vi "UHR-Fleezers Control (host) -Mau_stepping_gamma.vi"(0 "Tab Control":T5(tab)) -> ()   [LabVIEW 2013] (continued)
          frame #3 {
            # "Go to Bottom Dispensor"
            n244 = local read "Location Matrix"() -> (w465:string[][])
            n245 = Index Array(array=w465, index (row)=1) -> (element=w461:string[])  [unwired: 1 in]
            n246 = Decimate 1D Array(w461) -> (w459:string[], w457:string[], w455:string[])
            n247 = Concatenate Strings("1PA" ("Substring"), w459, "2PA" ("Substring"), w457, "3PA" ("Substring"), w455, "\r") -> (w463:string)
            n248 = local read "ESP Port"() -> (w462:refnum<visa-resource-name>)
            n249 = VISA Write(VISA resource name=w462, write buffer=w463) -> ()  [unwired: 1 in, 3 out]
          }
          frame #4 {
            n250 = Wait (ms)(milliseconds to wait=u32 200) -> ()  [unwired: 1 out]
          }
          frame #5 {
            # "Change the trajectory mode to Jog"
            n251 = local read "ESP Port"() -> (w467:refnum<visa-resource-name>)
            n252 = Concatenate Strings("1TJ3;\n2TJ3;\n3TJ3" ("Substring"), "\r") -> (w470:string)
            n253 = VISA Write(VISA resource name=w467, write buffer=w470) -> ()  [unwired: 1 in, 3 out]
          }
        }
      }
      event "Capture": Value Change {
        n254 = event-data() -> ()  [unwired: 1 in, 5 out]
        n255 = local read "Capture Locations"() -> (w471:i32)
        n256 = local read "Z Pos Pos"() -> (w472:string)
        n257 = local read "X Pos"() -> (w474:string)
        n258 = local read "Y Pos"() -> (w473:string)
        n259 = case shown="1" w471 {
          selector: w471 -> [w478 w485 w492 w499]
          tunnel: w474 -> [w481 w488 w495 w502]
          tunnel: w473 -> [w480 w487 w494 w501]
          tunnel: w472 -> [w479 w486 w493 w500]
          frame 0, Default {
            # "Capture Top Dispensor Location"
            n260 = local read "Location Matrix"() -> (w477:string[][])
            n261 = Build Array(w481, w480, w479) -> (w476:string[])
            n262 = Replace Array Subset(array=w477, new element=w476, index (row)=w478) -> (w475:string[][])  [unwired: 1 in]
            n263 = local write "Location Matrix"(w475) -> ()
          }
          frame 1 {
            # "Capture Bottom Dispensor Location"
            n264 = local read "Location Matrix"() -> (w484:string[][])
            n265 = Build Array(w488, w487, w486) -> (w483:string[])
            n266 = Replace Array Subset(array=w484, new element=w483, index (row)=w485) -> (w482:string[][])  [unwired: 1 in]
            n267 = local write "Location Matrix"(w482) -> ()
          }
          frame 2 {
            # "Capture Experimental Region Location"
            n268 = local read "Location Matrix"() -> (w491:string[][])
            n269 = Build Array(w495, w494, w493) -> (w490:string[])
            n270 = Replace Array Subset(array=w491, new element=w490, index (row)=w492) -> (w489:string[][])  [unwired: 1 in]
            n271 = local write "Location Matrix"(w489) -> ()
          }
          frame 3 {
            # "Capture Other Location"
            n272 = local read "Location Matrix"() -> (w498:string[][])
            n273 = Build Array(w502, w501, w500) -> (w497:string[])
            n274 = Replace Array Subset(array=w498, new element=w497, index (row)=w499) -> (w496:string[][])  [unwired: 1 in]
            n275 = local write "Location Matrix"(w496) -> ()
          }
        }
      }
      event "Save": Value Change {
        # "reshape Location Matrix to 1-D array to write"
        n276 = event-data() -> ()  [unwired: 1 in, 5 out]
        n277 = local read "Location Matrix"() -> (w506:string[][])
        n278 = local read "Location path"() -> (w503:path)
        n279 = Reshape Array(w506, 12) -> (w504:string[])
        n280 = Write to Text File(file (use dialog)=w503, text=w504) -> ()  [unwired: 2 in, 3 out]
      }
      event "Activate Joystick": Value Change {
        # "Change the trajectory mode to Jog"
        n281 = event-data() -> ()  [unwired: 1 in, 5 out]
        n282 = disable-structure shown="Disabled" {
          frame Disabled {
            n283 = case shown="True" "Activate Joystick" {
              frame False {
              }
              frame True {
                # "Change the trajectory mode to Jog"
                n284 = local read "ESP Port"() -> (w515:refnum<visa-resource-name>)
                n285 = Concatenate Strings("1TJ3;\n2TJ3;\n3TJ3" ("Substring"), "\r") -> (w512:string)
                n286 = VISA Write(VISA resource name=w515, write buffer=w512) -> ()  [unwired: 1 in, 3 out]
              }
            }
          }
          frame Enabled {
          }
        }
        n287 = local read "ESP Port"() -> (w507:refnum<visa-resource-name>)
        n288 = Concatenate Strings("1TJ3;\n2TJ3;\n3TJ3" ("Substring"), "\r") -> (w510:string)
        n289 = VISA Write(VISA resource name=w507, write buffer=w510) -> ()  [unwired: 1 in, 3 out]
      }
    }
  }
  n290 = disable-structure shown="Disabled" {
    disable-tunnel: w24 -> [w544 _]
    frame Disabled {
      w539 = T17 0 items=["Grayscale (U8)", "Grayscale (I16)", "Grayscale (SGL)", "Complex (CSG)", "RGB (U32)", "HSL (U32)", "RGB (U64)", "Grayscale (U16)"] ("Image Type")
      n291 = call <vilib>:"IMAQ Init.vi"("Interface Name"="img0") -> ("error out"=w541:errorcluster, "IMAQ Session Out"=w543:refnum<k11>)  [unwired: 9 in]
      n292 = call <vilib>:"IMAQ Grab Setup.vi"("error in (no error)"=w541, "IMAQ Session In"=w543) -> ("error out"=w537:errorcluster, "IMAQ Session Out"=w538:refnum<k11>)  [unwired: 8 in]
      n293 = call "IMAQ Create"("Image Name"="untitled", "Image Type"=w539) -> ("New Image"=w536:T3)  [unwired: 3 in, 1 out]
      n294 = call <vilib>:"Application Directory.vi"() -> ("Application Directory"=w523:path)
      n295 = Build Path(base path=w523, name or relative path="_trap_screen_positions") -> (appended path=w531:path)
      n296 = Open/Create/Replace File(file path (use dialog)=w531, operation (0:open)=T23."open or create", access (0:read/write)=enum16{"read/write", "read-only", "write-only"}."read/write") -> (refnum out=w533:refnum<file>)  [unwired: 3 in, 2 out]
      n297 = local read "Trap Sets"() -> (w525:u32)
      n298 = for "Load trap positions on video screen from file." {
        N: w525 -> [_]
        tunnel: [w551] -> w526
        tunnel: w533 -> [w550]
        tunnel: [w547] -> w522 mode=indexing
        w549 = 4
        n299 = for {
          N: w549 -> [_]
          tunnel: [w555] -> w551
          tunnel: w550 -> [w554]
          tunnel: w549 -> [w553]
          tunnel: [w552] -> w548 mode=indexing
          n300 = Read from Binary File(5:w553, 11:w554) -> (2:w552:i32, 3:w555:refnum<file>)  [unwired: 4 in, 2 out]
        }
        n301 = Array To Cluster(array=w548) -> (cluster=w547:T27)
      }
      n302 = node-c288() -> (w546:T24)  [unwired: 4 in]
      n303 = timed-loop "acquire video and stage position" {
        timing: w546 -> [_]
        timing-out: [_] -> w545
        tunnel: w538 -> [w574]
        tunnel: w537 -> [w573]
        tunnel: w536 -> [w572]
        tunnel: [w571] -> w518
        tunnel: [w568] -> w519
        tunnel: [w569] -> w517
        tunnel: w544 -> [_]
        shift-right: [w565] -> w535
        shift-left: w522 -> [w566]
        tunnel: w525 -> [w563]
        stop <- w570 stop-if-true
        n304 = node-c288() -> ()  [unwired: 1 in, 1 out]
        n305 = event shown="[0] Timeout" {
          selector: _ -> [_ _ _ _]
          dyn-events: _ -> [_ _ _ _]
          timeout: 10 -> [_ _ _ _]
          tunnel: w574 -> [w585 w600 w609 w628]
          tunnel: w573 -> [w584 w602 w607 w630]
          tunnel: w572 -> [w583 w601 w608 w629]
          tunnel: [w582 w600 w609 w628] -> w571
          tunnel: [w575 w604 FALSE FALSE] -> w570
          tunnel: [w579 w602 w607 w630] -> w569
          tunnel: [w578 w601 w608 w629] -> w568
          tunnel: "radius" -> [_ _ w614 _]
          tunnel: w566 -> [w576 w603 w612 _]
          tunnel: [w576 w603 w613 cluster{i32, i32, i32, i32}[] []] -> w565
          tunnel: w563 -> [_ _ w605 _]
          event Timeout {
            n306 = event-data() -> ()  [unwired: 1 in, 2 out]
            n307 = call <vilib>:"IMAQ Grab Acquire.vi"("error in (no error)"=w584, "Image In"=w583, "IMAQ Session In"=w585) -> ("error out"=w580:errorcluster, "Image Out"=w581:T3, "IMAQ Session Out"=w582:refnum<k11>)  [unwired: 5 in, 1 out]
            n308 = case shown="True" "trap\nmarkers?" {
              tunnel: w576 -> [_ w593]
              tunnel: w581 -> [w587 w592]
              tunnel: w580 -> [w586 w591]
              tunnel: [w586 w590] -> w579
              tunnel: [w587 w588] -> w578
              frame False {
              }
              frame True {
                n309 = for {
                  tunnel: w593 -> [w599] mode=indexing
                  shift-right: [w597] -> w588
                  shift-left: w592 -> [w598]
                  tunnel: w591 -> [w596]
                  tunnel: [w595] -> w590
                  tunnel: u32 16711680 ("Color") -> [w594]
                  n310 = call "IMAQ Overlay Oval"("Color"=w594, "error in (no error)"=w596, "Bounding Rectangle"=w599, "Image"=w598) -> ("error out"=w595:errorcluster, "Image Out"=w597:T3)  [unwired: 6 in]
                }
              }
            }
            "Primary Video Display" <- w578
            n311 = Unbundle By Name(w580) -> ("status"=w575:bool)
          }
          event "Stop All": Value Change {
            n312 = event-data() -> ()  [unwired: 1 in, 5 out]
            n313 = local read "Stop All"() -> (w604:bool)
          }
          event "Primary Video Display": Mouse Down {
            n314 = event-data() -> ()  [unwired: 1 in, 7 out]
            n315 = Array Size(array=w612) -> (size(s)=w611:i32)
            n316 = Less?(x=w611, y=w605) -> (x < y?=w610:bool)
            n317 = case shown="True" w610 {
              tunnel: w614 -> [_ w624]
              tunnel: w612 -> [w615 w618]
              tunnel: [w615 w617] -> w613
              frame False {
              }
              frame True {
                n318 = property on="Primary Video Display" class="ImageControl"() -> ("Last Mouse Position"=w616:cluster{"X":i32, "Y":i32})  [unwired: 2 in, 2 out]
                n319 = Unbundle By Name(w616) -> ("X"=w626:i32, "Y"=w625:i32)
                n320 = Add(x=w625, y=w624) -> (x+y=w622:i32)
                n321 = Subtract(x=w625, y=w624) -> (x-y=w620:i32)
                n322 = Add(x=w626, y=w624) -> (x+y=w621:i32)
                n323 = Subtract(x=w626, y=w624) -> (x-y=w623:i32)
                n324 = Bundle(w623, w622, w621, w620) -> (w619:cluster{i32, i32, i32, i32})  [unwired: 1 in]
                n325 = Build Array (concatenate)(w618, w619) -> (w617:T28)
              }
            }
          }
          event "clear markers": Value Change {
            n326 = event-data() -> ()  [unwired: 1 in, 5 out]
          }
        }
        n327 = node-c288() -> ()  [unwired: 1 in, 1 out]
      }
      n328 = node-c288(w545) -> ()  [unwired: 1 out]
      n329 = Set File Position(offset (in bytes) (0)=i64 0, refnum=w526, from (0:start)=enum16{"start", "end", "current"}."start") -> (refnum out=w527:refnum<file>)  [unwired: 1 in, 1 out]
      n330 = for "Write trap positions to file so they can be remembered\nwhen program is removed from memory" {
        tunnel: w535 -> [w559] mode=indexing
        tunnel: [w557] -> w534
        tunnel: w527 -> [w556]
        n331 = Cluster To Array(cluster=w559) -> (array=w558:i32[])
        n332 = for {
          tunnel: w558 -> [w562] mode=indexing
          tunnel: [w561] -> w557
          tunnel: w556 -> [w560]
          n333 = Write to Binary File(file (use dialog)=w560, data=w562) -> (refnum out=w561:refnum<file>)  [unwired: 4 in, 2 out]
        }
      }
      n334 = Close File(refnum=w534) -> ()  [unwired: 1 in, 2 out]
      n335 = call "IMAQ Dispose"("Image"=w519, "error in (no error)"=w517) -> ("error out"=w516:errorcluster)  [unwired: 4 in]
      n336 = call <vilib>:"IMAQ Stop.vi"("error in (no error)"=w516, "IMAQ Session In"=w518) -> ("error out"=w520:errorcluster, "IMAQ Session Out"=w521:refnum<k11>)  [unwired: 8 in]
      n337 = call <vilib>:"IMAQ Close.vi"("error in (no error)"=w520, "IMAQ Session In"=w521) -> ()  [unwired: 9 in, 1 out]
    }
    frame Enabled {
    }
  }
  n338 = disable-structure shown="Enabled" {
    disable-tunnel: [w637 _] -> w35
    disable-tunnel: w24 -> [w636 _]
    frame Enabled {
      n339 = node-c288() -> (w639:T24)  [unwired: 4 out]
      n340 = timed-loop "Rough control of MCL mirror stage (debugging)" {
        tunnel: w636 -> [w642]
        tunnel: [w641] -> w637
        timing: w639 -> [_]
        timing-out: [_] -> w638
        stop <- w641 stop-if-true
        n341 = node-c288() -> ()  [unwired: 2 out]
        n342 = case shown="1" "MCL Mode" {
          tunnel: w642 -> [_ w645 w692]
          frame 0, Default {
            # "manual positioning"
          }
          frame 1 {
            # "sinusoidal wave"
            n343 = node-c288() -> (w647:T24)  [unwired: 4 out]
            n344 = timed-loop "Oscillate MCL mirror" {
              timing: w647 -> [_]
              timing-out: [_] -> w646
              tunnel: w645 -> [w686]
              i -> [w685]
              stop <- w648 stop-if-true
              n345 = node-c288() -> (w684:i64)  [unwired: 1 out]
              n346 = Multiply(x="AO1", y=32767.0) -> (x*y=w680:dbl)
              n347 = Multiply(x="AO2", y=32767.0) -> (x*y=w675:dbl)
              n348 = Divide(x=w680, y=10.0) -> (x/y=w681:dbl)
              n349 = Divide(x=w675, y=10.0) -> (x/y=w676:dbl)
              n350 = To Word Integer(number=w681) -> (16bit integer=w673:i16)
              n351 = To Word Integer(number=w676) -> (16bit integer=w672:i16)
              n352 = Divide(x=w684, y=i64 1000) -> (x/y=w655:dbl)
              n353 = Multiply(x=w655, y=w685) -> (x*y=w666:dbl)
              n354 = Multiply(x="Osc. freq. (Hz) 2", y=6.283185307179586) -> (x*y=w667:dbl)
              n355 = Multiply(x=w667, y=w666) -> (x*y=w665:dbl)
              n356 = Sine(x=w665) -> (sin(x)=w664:dbl)
              n357 = Multiply(x=w664, y="Osc. amp. (V)") -> (x*y=w662:dbl)
              n358 = Add(x=w662, y="Osc. center (V)") -> (x+y=w660:dbl)
              n359 = Divide(x=w660, y=10.0) -> (x/y=w658:dbl)
              n360 = Multiply(x=w658, y=32767.0) -> (x*y=w653:dbl)
              n361 = Select(t=w653, s="Scan axis", f=w673) -> (s? t:f=w671:dbl)
              n362 = Select(t=w672, s="Scan axis", f=w653) -> (s? t:f=w670:dbl)
              n363 = local read "MCL Mode"() -> (w652:u16)
              n364 = Not Equal?(x=w652, y=u16 1) -> (x != y?=w649:bool)
              n365 = local read "Stop All"() -> (w650:bool)
              n366 = xnode "Read/Write Control"("FPGA VI Reference In"=w686, "AO1"=w671, "AO2"=w670) -> ()  [unwired: 1 in, 2 out]
              n367 = Compound Arithmetic op=OR(w650, w649) -> (w648:bool)
              n368 = node-c288() -> ()  [unwired: 2 out]
            }
            n369 = node-c288(w646) -> ()  [unwired: 1 out]
          }
          frame 2 {
            # "linear scan"
            n370 = case shown="True" "Start Scan" {
              tunnel: w692 -> [_ w704]
              frame False {
              }
              frame True {
                n371 = Subtract(x="End (V)", y="Begin (V)") -> (x-y=w700:dbl)
                n372 = Decrement(x="N Points") -> (x-1=w699:dbl)
                n373 = Divide(x=w700, y=w699) -> (x/y=w697:dbl)
                n374 = for {
                  N: "N Points" -> [_]
                  tunnel: "Begin (V)" -> [w717]
                  tunnel: w704 -> [w709]
                  tunnel: [w708] -> w703 mode=indexing
                  tunnel: w697 -> [w707]
                  tunnel: [w705] -> w696 mode=indexing
                  i -> [w716]
                  n375 = Multiply(x=w707, y=w716) -> (x*y=w715:dbl)
                  n376 = Add(x=w717, y=w715) -> (x+y=w712:dbl)
                  n377 = local read "Scan axis"() -> (w706:bool)
                  n378 = local read "AO1"() -> (w714:dbl)
                  n379 = local read "AO2"() -> (w713:dbl)
                  n380 = Select(t=w712, s=w706, f=w714) -> (s? t:f=w711:dbl)
                  n381 = Select(t=w713, s=w706, f=w712) -> (s? t:f=w710:dbl)
                  n382 = flat-sequence {
                    tunnel: w711 -> [w721]
                    tunnel: w710 -> [w720]
                    tunnel: w709 -> [w718]
                    tunnel: [w731] -> w708
                    tunnel: [w730] -> w705
                    frame #0 {
                      w724 = 10.0 ("y")
                      w719 = 32767.0 ("y")
                      n383 = Multiply(x=w721, y=w719) -> (x*y=w727:dbl)
                      n384 = Multiply(x=w720, y=w719) -> (x*y=w725:dbl)
                      n385 = Divide(x=w727, y=w724) -> (x/y=w728:dbl)
                      n386 = Divide(x=w725, y=w724) -> (x/y=w726:dbl)
                      n387 = To Word Integer(number=w728) -> (16bit integer=w722:i16)
                      n388 = To Word Integer(number=w726) -> (16bit integer=w723:i16)
                      n389 = xnode "Read/Write Control"("FPGA VI Reference In"=w718, "AO1"=w722, "AO2"=w723) -> ()  [unwired: 1 in, 2 out]
                    }
                    frame #1 {
                      n390 = Wait (ms)(milliseconds to wait="DAQ Delay (ms)") -> ()  [unwired: 1 out]
                    }
                    frame #2 {
                      n391 = local read "Slow mean"() -> (w731:dbl)
                      n392 = local read "Sigma"() -> (w730:dbl)
                    }
                  }
                }
                n393 = Bundle("Begin (V)"="Begin (V)", w697, w703) -> (→"MCL Scan":cluster{"Begin (V)":dbl, dbl, dbl[]})  [unwired: 1 out]
                n394 = Bundle("Begin (V)"="Begin (V)", w697, w696) -> (→"MCL Scan 2":cluster{"Begin (V)":dbl, dbl, dbl[]})  [unwired: 1 out]
              }
            }
          }
        }
        n395 = local read "Stop All"() -> (w641:bool)
        n396 = node-c288() -> ()  [unwired: 2 out]
      }
      n397 = node-c288(w638) -> ()  [unwired: 1 out]
    }
    frame Disabled {
    }
  }
  n398 = node-c288(2 ("Processor")) -> (w15:T24)  [unwired: 3 in]
  n399 = node-c288() -> (w69:T24)  [unwired: 4 in]
  n400 = timed-loop "Control parameters (event loop)" {
    tunnel: w24 -> [w737]
    shift-right: [w736] -> _
    shift-left: errorcluster {"status"=FALSE, "code"=0, "source"=""} ("error out") -> [w735]
    tunnel: [w734] -> w37
    timing: w15 -> [_]
    timing-out: [_] -> w14
    stop <- w734 stop-if-true
    n401 = node-c288() -> ()  [unwired: 1 in, 1 out]
    n402 = event shown="[7] \"Simulate motor gamma distribution\": Value Change" {
      selector: _ -> [_ _ _ _ _ _ _ _ _ _ _ _ _ _ _ _ _ _ _ _ _ _ _ _ _ _ _ _ _ _ _ _ _ _ _ _ _ _ _ _ _ _ _ _ _ _ _ _ _ _ _ _ _ _ _ _ _]
      dyn-events: _ -> [_ _ _ _ _ _ _ _ _ _ _ _ _ _ _ _ _ _ _ _ _ _ _ _ _ _ _ _ _ _ _ _ _ _ _ _ _ _ _ _ _ _ _ _ _ _ _ _ _ _ _ _ _ _ _ _ _]
      timeout: _ -> [_ _ _ _ _ _ _ _ _ _ _ _ _ _ _ _ _ _ _ _ _ _ _ _ _ _ _ _ _ _ _ _ _ _ _ _ _ _ _ _ _ _ _ _ _ _ _ _ _ _ _ _ _ _ _ _ _]
      tunnel: w737 -> [w775 _ _ _ w812 _ w834 w864 _ w951 _ _ _ w994 _ _ w1037 w1043 w1048 w1054 w1090 w1108 w1115 w1133 w1144 w1155 w1166 w1177 w1188 w1206 w1212 w1306 _ w1315 w1353 _ w1388 w1392 w1403 w1407 w1411 _ w1419 _ _ _ _ _ w1555 _ w1572 w1575 w1584 w1587 w1591 _ w1608]
      tunnel: [w774 _ _ _ w802 _ w833 w863 _ w914 _ w959 _ w973 _ _ w1036 w1039 w1045 w1051 w1089 w1106 w1114 w1127 w1138 w1149 w1160 w1171 w1182 w1204 w1211 w1304 _ w1313 w1351 _ w1386 w1390 w1393 w1405 w1409 _ w1417 _ _ _ _ _ w1553 _ _ _ _ _ _ _ _] -> w736
      tunnel: w735 -> [w773 _ _ _ w811 _ w832 w862 _ w946 _ w959 _ w993 _ _ w1035 w1038 w1044 w1050 w1088 w1107 w1113 w1132 w1143 w1154 w1165 w1176 w1187 w1205 w1210 w1305 _ w1314 w1352 _ w1387 w1391 w1402 w1406 w1410 _ w1418 _ _ _ _ _ w1554 _ w1571 w1574 w1583 w1586 w1590 _ w1607]
      tunnel: [_ _ _ _ _ _ _ _ _ _ _ w958 _ _ _ _ _ _ _ _ _ _ _ _ _ _ _ _ _ _ _ _ _ _ _ _ _ _ _ _ _ _ _ _ _ _ _ _ _ _ _ _ _ _ _ _ _] -> w734
      tunnel: [_ _ _ _ _ _ _ _ "Round T1 X" _ _ _ _ _ _ _ _ _ _ _ _ _ _ _ _ _ _ _ _ _ _ _ _ _ _ _ _ _ _ _ _ _ _ _ _ _ _ _ _ _ _ _ _ _ _ _ _] -> _
      tunnel: [_ _ _ "Adjust Scale\nto Mean" _ _ _ _ _ _ _ _ _ _ _ _ _ _ _ _ _ _ _ _ _ _ _ _ _ _ _ _ _ _ _ _ _ _ _ _ _ _ _ _ _ _ _ _ _ _ _ _ _ _ "Set SP to Reading" _ _] -> _
      tunnel: [_ _ _ _ _ _ _ _ _ _ "Round T2 X" _ "Delayed Interlace Start" _ _ _ _ _ _ _ _ _ _ _ _ _ _ _ _ _ _ _ _ _ _ _ _ _ _ _ _ _ _ _ _ _ _ _ _ _ _ _ _ _ _ _ _] -> _
      event "AI Count (ticks)", "Sets to FIFO (Traps)", "Save ave N", "FPGA Ave.", "# Samples/channel", "N sets to save": Value Change {
        # "So that if 'Save ave N' is updated, the AOD scanning code updates too."
        n403 = event-data() -> ()  [unwired: 6 out]
        n404 = local read "AI Count (ticks)"() -> (w755:u32)
        n405 = Boolean To (0,1)(Boolean="Sets to FIFO (Traps)") -> (0, 1=w765:cluster{"Set 1":i16, "Set 2":i16, "Set 3":i16})
        n406 = xnode "Read/Write Control"("FPGA VI Reference In"=w775, "error in"=w773, "ai count"=w755, "AI1 Sets to FIFO"="Sets to FIFO (Traps)", "N of AI1 Int Acq Sets"="N Acq Sets (Traps + Fl.)") -> ("error out"=w774:errorcluster)  [unwired: 1 out]
        n407 = Cluster To Array(cluster=w765) -> (array=w764:i16[])
        n408 = To Unsigned Long Integer(number=w764) -> (unsigned 32bit integer=w744:u32[])
        n409 = local read "Scan steps (AOD)"() -> (w766:u64)
        n410 = Multiply(x=w755, y="N Acq Sets (Traps + Fl.)") -> (x*y=w753:u32)
        n411 = Divide(x=40000000.0, y=w755) -> (x/y=w747:dbl)
        "AI rate (Hz)" <- w747
        "Ave. Rate (Hz)" <- w747
        n412 = Add Array Elements(numeric array=w744) -> (sum=w756:u32)
        "Trap Sets" <- w756
        n413 = Reciprocal(x=w747) -> (1/x=→"Ave. Period (s)":dbl)
        n414 = property on="Scan steps (AOD)" class="DigNum (strict)"("Val(Sgnl)"=w766) -> ()  [unwired: 2 in, 2 out]
        n415 = Divide(x=w747, y="N Acq Sets (Traps + Fl.)") -> (x/y=w770:dbl)
        "Data Rate (Hz)" <- w770
        n416 = Reciprocal(x=w770) -> (1/x=→"Data Period (s)":dbl)
        n417 = local read "Save ave N"() -> (w769:dbl)
        n418 = Divide(x=w770, y=w769) -> (x/y=w768:dbl)
        "Save Data Rate (Hz)" <- w768
        n419 = Reciprocal(x=w768) -> (1/x=→"Save Data Period (s)":dbl)
        n420 = Multiply(x=w753, y="# Samples/trap") -> (x*y=w751:u32)
        "Counts/DMA" <- w751
        n421 = property on="Trap Disp. Downsample" class="DigNum (strict)"("Maximum"="# Samples/trap") -> ()  [unwired: 2 in, 2 out]
        n422 = Multiply(x=w756, y="# Samples/trap") -> (x*y=w745:u32)
        "# Samples/channel" <- w745
        n423 = Multiply(x=w745, y=u32 8) -> (x*y=→"Trap AI Elements/DMA read":u32)
        n424 = local read "APD Int. Count"() -> (w752:u32)
        n425 = Multiply(x=w745, y=u32 3) -> (x*y=→"Trap Pos Elements/DMA read":u32)
        n426 = Divide(x=w751, y=w752) -> (x/y=w742:dbl)
        "APD Samples/FIFO Acq." <- w742
        n427 = Divide(x=w751, y=40000000.0) -> (x/y=w749:dbl)
        "DMA Update Period (s)" <- w749
        n428 = Multiply(x=2.0, y=w742) -> (x*y=→"APD Elements/DMA read":dbl)
        n429 = property on="APD Disp. Downsample" class="DigNum (strict)"("Maximum"=w742) -> ()  [unwired: 2 in, 2 out]
        n430 = local read "N sets to save"() -> (w762:u32)
        n431 = Multiply(x=w749, y=w762) -> (x*y=→"Total Time (s)":dbl)
        "FPGA Averaging" <- FALSE ("FPGA Averaging")
      }
      event "Rescale on Mean": Value Change {
        n432 = event-data() -> ()  [unwired: 7 out]
        n433 = And(x=FALSE, y="Rescale on Mean") -> (x .and. y?=w777:bool)
        n434 = local write "Rescale on Mean"(w777) -> ()
        n435 = local read "Bead Mean (nm)"() -> (w782:dbl)
        n436 = Add(x="Amplitude (nm)", y=w782) -> (x+y=w780:dbl)
        n437 = Subtract(x=w782, y="Amplitude (nm)") -> (x-y=w779:dbl)
        n438 = property on="Bead Separation" class="WFChart (strict)"("YScale.Minimum"=w779) -> ()  [unwired: 2 in, 2 out]
        n439 = property on="Bead Separation" class="WFChart (strict)"("YScale.Maximum"=w780) -> ()  [unwired: 2 in, 2 out]
      }
      event "Detector Type": Value Change {
        n440 = event-data() -> ()  [unwired: 7 out]
        n441 = local read "AI labels"() -> (w783:string[])
        n442 = property on="High Res. Display" class="Ring (strict)"("Strings []"=w783) -> ()  [unwired: 2 in, 2 out]
        n443 = Build Array (concatenate)(w783, "none") -> (w784:string[])
        n444 = property on="FFT 1 Choice 1" class="Ring (strict)"("Strings []"=w784) -> ()  [unwired: 2 in, 2 out]
        n445 = property on="FFT 1 Choice 2" class="Ring (strict)"("Strings []"=w784) -> ()  [unwired: 2 in, 2 out]
        n446 = property on="FFT 2 Choice 1" class="Ring (strict)"("Strings []"=w784) -> ()  [unwired: 2 in, 2 out]
        n447 = property on="FFT 2 Choice 2" class="Ring (strict)"("Strings []"=w784) -> ()  [unwired: 2 in, 2 out]
        n448 = Bundle("APD 1", "APD 2") -> (w787:cluster{string, string})  [unwired: 1 out]
        n449 = Cluster To Array(cluster=w787) -> (array=w785:string[])
        n450 = Build Array (concatenate)(w785, w784) -> (w789:string[])
        n451 = Array Size(array=w789) -> (size(s)=w790:i32)
        n452 = property on="Signals to Plot" class="LstBox (strict)"("Item Names"=w789) -> ()  [unwired: 2 in, 2 out]
        n453 = property on="Signals to Plot" class="LstBox (strict)"("Number of Rows"=w790) -> ()  [unwired: 2 in, 2 out]
        n454 = property on="All Signals" class="WFChart (strict)"("LegNumRows"=w790) -> ()  [unwired: 2 in, 2 out]
      }
      event "Adjust Scale\nto Mean": Value Change {
        n455 = event-data() -> ()  [unwired: 7 out]
        n456 = local read "APD 1 Rate (Hz)"() -> (w799:dbl)
        n457 = Multiply(x=1000.0, y="Above (kHz)") -> (x*y=w797:dbl)
        n458 = Multiply(x=1000.0, y="Below (kHz)") -> (x*y=w795:dbl)
        n459 = Add(x=w797, y=w799) -> (x+y=w792:dbl)
        n460 = Subtract(x=w799, y=w795) -> (x-y=w793:dbl)
        n461 = property on="APD Chart" class="WFChart (strict)"("YScale.Minimum"=w793) -> ()  [unwired: 2 in, 2 out]
        n462 = property on="APD Chart" class="WFChart (strict)"("YScale.Maximum"=w792) -> ()  [unwired: 2 in, 2 out]
      }
      event "Phase adj. (AI1)", "+ phase (AI1)", "- phase (AI1)": Value Change {
        n463 = event-data() -> ()  [unwired: 7 out]
        n464 = Negate(x="Phase adj. (AI1)") -> (-x=w809:i16)
        n465 = Select(t=w809, s="- phase (AI1)", f="Phase adj. (AI1)") -> (s? t:f=w808:i16)
        n466 = xnode "Read/Write Control"("FPGA VI Reference In"=w812, "error in"=w811, "Phase count adjustment"=w808) -> ("FPGA VI Reference Out"=w807:T19, "error out"=w806:errorcluster)
        n467 = Or(x="- phase (AI1)", y="+ phase (AI1)") -> (x .or. y?=w803:bool)
        n468 = xnode "Read/Write Control"("FPGA VI Reference In"=w807, "error in"=w806, "+ phase"=w803) -> ("error out"=w802:errorcluster)  [unwired: 1 out]
      }
      event "Signals to Plot": Double Click {
        w815 = u32 9868950 ("Color Box")
        n469 = event-data() -> ("Row"=w817:i32)  [unwired: 9 out]
        n470 = property on="All Signals" class="WFChart (strict)"("Active Plot"=w817) -> (error out=w828:errorcluster)  [unwired: 2 in, 1 out]
        n471 = property on="All Signals" class="WFChart (strict)" props=["Plot", "Visible?", "Plot", "Plot Color"](error in=w828) -> (error out=w827:errorcluster, "Plot.Visible?"=w826:bool)  [unwired: 1 in, 2 out]
        n472 = Select(t=FALSE ("Plot.Visible"), s=w826, f=TRUE ("Plot.Visible")) -> (s? t:f=w821:bool)
        n473 = property on="All Signals" class="WFChart (strict)"(error in=w827, "Plot.Visible?"=w821) -> (error out=w823:errorcluster)  [unwired: 1 in, 1 out]
        n474 = property on="All Signals" class="WFChart (strict)"(error in=w823) -> (error out=w818:errorcluster, "Plot.Plot Color"=w822:u32)  [unwired: 1 in, 1 out]
        n475 = property on="Signals to Plot" class="LstBox (strict)"(error in=w818, "Active Row"=w817) -> (error out=w816:errorcluster)  [unwired: 1 in, 1 out]
        n476 = Select(t=w822, s=w821, f=u32 0) -> (s? t:f=w819:u32)
        n477 = property on="Signals to Plot" class="LstBox (strict)"(error in=w816, "CellFontColor"=w819, "SelColor"=w815, "CellBG"=w815, "CellFontSize"=u32 20 ("Active Row:Cell Font:Size"), "CellFontBold"=TRUE ("Active Row:Cell Font:Bold")) -> ()  [unwired: 1 in, 2 out]
      }
      event "BD 1 Frequency 1 (MHz)", "BD 1 Frequency 2 (MHz)", "BD 1 Frequency 3 (MHz)", "BD 2 Frequency 1 (MHz)", "BD 2 Frequency 2 (MHz)", "BD 2 Frequency 3 (MHz)", "Trap Delta (MHz)": Value Change {
        # "anytime one of the frequencies is changed, write it to the RF board UNLESS Set 2 is being oscillated. The oscillation\nscript writes the frequencies to the RF board."
        n478 = event-data() -> ("CtlRef"=w831:refnum<vi>)  [unwired: 6 out]
        n479 = control-ref of="Trap Delta (MHz)"() -> (w830:refnum<vi>)
        n480 = Equal?(x=w830, y=w831) -> (x = y?=w829:bool)
        n481 = case shown="False" "Oscillate Set 2" {
          tunnel: w834 -> [w857 _]
          tunnel: [w856 w860] -> w833
          tunnel: w832 -> [w855 w860]
          tunnel: w829 -> [w842 _]
          frame False {
            w836 = 80
            n482 = local read "BD 1 Frequency 2 (MHz)"() -> (w844:dbl)
            n483 = Divide(x="Trap Delta (MHz)", y=2) -> (x/y=w838:dbl)
            n484 = Subtract(x=w836, y=w838) -> (x-y=w837:dbl)
            n485 = local write "BD 1 Frequency 1 (MHz)"(w837) -> ()
            n486 = Add(x=w836, y=w838) -> (x+y=w843:dbl)
            n487 = Select(t=w843, s=w842, f=w844) -> (s? t:f=w841:dbl)
            n488 = local read "Y RF Frequency Limits (MHz)"() -> (w845:T16)
            n489 = local read "X RF Frequency Limits (MHz)"() -> (w846:T16)
            n490 = local read "BD 1 Frequency 3 (MHz)"() -> (w858:dbl)
            n491 = local write "BD 1 Frequency 2 (MHz)"(w841) -> ()
            n492 = local read "BD 2 Frequency 1 (MHz)"() -> (w849:dbl)
            n493 = local read "BD 2 Frequency 2 (MHz)"() -> (w848:dbl)
            n494 = local read "BD 2 Frequency 3 (MHz)"() -> (w859:dbl)
            n495 = call "set RF board frequency - interlace.vi"("Board 2 Frequency Limits"=w845, "Board 1 Frequency Limits"=w846, "error in"=w855, "FPGA VI Reference In"=w857, "Board 2 Frequency 3 (MHz)"=w859, "Board 1 Frequency 3 (MHz)"=w858, "Board 2 Frequency 2 (MHz)"=w848, "Board 2 Frequency 1 (MHz)"=w849, "Board 1 Frequency 2 (MHz)"=w841, "Board 1 Frequency 1  (MHz)"=w837) -> ("error out"=w856:errorcluster)  [unwired: 1 out]
            n496 = Subtract(x=w849, y=w848) -> (x-y=w853:dbl)
            n497 = Subtract(x=w841, y=w837) -> (x-y=w854:dbl)
            n498 = Square(x=w853) -> (x^2=w851:dbl)
            n499 = Square(x=w854) -> (x^2=w852:dbl)
            n500 = Add(x=w852, y=w851) -> (x+y=w850:dbl)
            n501 = Square Root(x=w850) -> (sqrt(x)=w847:dbl)
            n502 = local write "Trap Delta (MHz)"(w847) -> ()
            n503 = property on="Initial delta (MHz)" class="DigNum (strict)"("Val(Sgnl)"=w847) -> ()  [unwired: 2 in, 2 out]
          }
          frame True {
          }
        }
      }
      event "Simulate motor gamma distribution": Value Change {
        n504 = event-data() -> ()  [unwired: 7 out]
        n505 = flat-sequence {
          tunnel: w864 -> [w867]
          tunnel: w862 -> [w865]
          tunnel: [w866] -> w861
          tunnel: [w910] -> w863
          tunnel: w861 -> [w910]
          frame #0 {
            n506 = while {
              tunnel: w867 -> [w908]
              tunnel: [w907] -> w866
              tunnel: w865 -> [w906]
              i -> [w890]
              stop <- w892 stop-if-true
              n507 = Divide(x="Backtrack probability", y=100) -> (x/y=w883:dbl)
              n508 = Random Number (0-1)() -> (number: 0 to 1=w882:dbl)
              n509 = Greater?(x=w882, y=w883) -> (0:w881:bool)
              n510 = Select(t=1, s=w881, f=-1) -> (s? t:f=w878:i32)
              n511 = local read "BD 1 Frequency 2 (MHz)"() -> (w894:dbl)
              n512 = Multiply(x=w878, y="Step size (nm)") -> (x*y=w876:dbl)
              "Step taken (nm)" <- w876
              n513 = Divide(x=w876, y=168.33) -> (x/y=w874:dbl)
              n514 = local read "BD 1 Frequency 1 (MHz)"() -> (w895:dbl)
              n515 = Add(x=w894, y=w874) -> (x+y=w893:dbl)
              n516 = local read "Y RF Frequency Limits (MHz)"() -> (w896:T16)
              n517 = local read "X RF Frequency Limits (MHz)"() -> (w897:T16)
              n518 = local write "BD 1 Frequency 2 (MHz)"(w893) -> ()
              n519 = local read "BD 2 Frequency 1 (MHz)"() -> (w900:dbl)
              n520 = local read "BD 2 Frequency 2 (MHz)"() -> (w899:dbl)
              n521 = call "set RF board frequency - interlace.vi"("Board 2 Frequency Limits"=w896, "Board 1 Frequency Limits"=w897, "error in"=w906, "FPGA VI Reference In"=w908, "Board 2 Frequency 2 (MHz)"=w899, "Board 2 Frequency 1 (MHz)"=w900, "Board 1 Frequency 2 (MHz)"=w893, "Board 1 Frequency 1  (MHz)"=w895) -> ("error out"=w907:errorcluster)  [unwired: 2 in, 1 out]
              n522 = Subtract(x=w900, y=w899) -> (x-y=w904:dbl)
              n523 = Subtract(x=w893, y=w895) -> (x-y=w905:dbl)
              n524 = Square(x=w904) -> (x^2=w902:dbl)
              n525 = Square(x=w905) -> (x^2=w903:dbl)
              n526 = Add(x=w903, y=w902) -> (x+y=w901:dbl)
              n527 = Square Root(x=w901) -> (sqrt(x)=w898:dbl)
              n528 = local write "Trap Delta (MHz)"(w898) -> ()
              n529 = property on="Initial delta (MHz)" class="DigNum (strict)"("Val(Sgnl)"=w898) -> ()  [unwired: 2 in, 2 out]
              n530 = call-poly <vilib>:"Continuous Random.vi"("c"="Shape", "b"="Scale parameter (s)", "samples"=1) -> ("gamma random numbers"=w873:dbl[])  [unwired: 7 in, 1 out]
              n531 = Index Array(array=w873) -> (element=w870:dbl)  [unwired: 1 in]
              "Dwell time (s)" <- w870
              n532 = Multiply(x=w870, y=1000) -> (x*y=w872:dbl)
              n533 = Add(x=w890, y=1) -> (x+y=w888:i32)
              n534 = To Unsigned Long Integer(number=w872) -> (unsigned 32bit integer=w871:u32)
              n535 = Wait (ms)(milliseconds to wait=w871) -> ()  [unwired: 1 out]
              n536 = Equal?(x=w888, y="Steps number") -> (x = y?=w892:bool)
            }
          }
          frame #1 {
            n537 = local write "Simulate motor gamma distribution"(FALSE) -> ()
          }
        }
      }
      event "Round T1 X": Value Change {
        n538 = event-data() -> ()  [unwired: 7 out]
        n539 = local read "BD 1 Frequency 1 (MHz)"() -> (w913:dbl)
        n540 = Round To Nearest(number=w913) -> (nearest integer value=w912:dbl)
        n541 = property on="BD 1 Frequency 1 (MHz)" class="DigNum (strict)"("Val(Sgnl)"=w912) -> ()  [unwired: 2 in, 2 out]
      }
      event "Restart RF": Value Change {
        n542 = event-data() -> ()  [unwired: 7 out]
        n543 = xnode "Read/Write Control"("FPGA VI Reference In"=w951, "error in"=w946, "FPGA Controls  RF Box"=FALSE) -> ("FPGA VI Reference Out"=w950:T19, "error out"=w945:errorcluster)
        n544 = local read "Y RF Amplitude Limits (%)"() -> (w926:T16)
        n545 = local read "X RF Amplitude Limits (%)"() -> (w927:T16)
        n546 = local read "X RF Frequency Limits (MHz)"() -> (w929:T16)
        n547 = local read "Y RF Frequency Limits (MHz)"() -> (w928:T16)
        n548 = xnode "Read/Write Control"("FPGA VI Reference In"=w950, "error in"=w945, "Direct RF Box  Communication"=TRUE) -> ("FPGA VI Reference Out"=w949:T19, "error out"=w944:errorcluster)
        n549 = local read "BD 2 Frequency 3 (MHz)"() -> (w936:dbl)
        n550 = local read "BD 2 Frequency 2 (MHz)"() -> (w937:dbl)
        n551 = local read "BD 1 Frequency 3 (MHz)"() -> (w940:dbl)
        n552 = local read "BD 1 Frequency 1 (MHz)"() -> (w941:dbl)
        n553 = local read "BD 2 Frequency 1 (MHz)"() -> (w938:dbl)
        n554 = local read "BD 1 Frequency 2 (MHz)"() -> (w939:dbl)
        n555 = call "Initialize RF boards - interlace 3.vi"("error in"=w944, "FPGA VI Reference In"=w949) -> ("error out"=w943:errorcluster, "FPGA VI Reference Out"=w948:T19)
        n556 = local read "BD 2 Amplitude 2 (%)"() -> (w931:dbl)
        n557 = local read "BD 2 Amplitude 1 (%)"() -> (w932:dbl)
        n558 = local read "BD 2 Amplitude 3 (%)"() -> (w930:dbl)
        n559 = local read "BD 1 Amplitude 3 (%)"() -> (w935:dbl)
        n560 = local read "BD 1 Amplitude 1 (%)"() -> (w934:dbl)
        n561 = local read "BD 1 Amplitude 2 (%)"() -> (w933:dbl)
        n562 = call "set RF board frequency - interlace.vi"("Board 2 Frequency Limits"=w928, "Board 1 Frequency Limits"=w929, "error in"=w943, "FPGA VI Reference In"=w948, "Board 2 Frequency 3 (MHz)"=w936, "Board 1 Frequency 3 (MHz)"=w940, "Board 2 Frequency 2 (MHz)"=w937, "Board 2 Frequency 1 (MHz)"=w938, "Board 1 Frequency 2 (MHz)"=w939, "Board 1 Frequency 1  (MHz)"=w941) -> ("error out"=w942:errorcluster, "FPGA VI Reference Out"=w947:T19)
        n563 = call "set RF board amplitude - interlace.vi"("Board 2 Amplitude Limits"=w926, "Board 1 Amplitude Limits"=w927, "error in"=w942, "FPGA VI Reference In"=w947, "Board 2 Amplitude 3 (%)"=w930, "Board 1 Amplitude 3 (%)"=w935, "Board 2 Amplitude 2 (%)"=w931, "Board 2 Amplitude 1 (%)"=w932, "Board 1 Amplitude 2 (%)"=w933, "Board 1 Amplitude 1 (%)"=w934) -> ("error out"=w919:errorcluster, "FPGA VI Reference Out"=w923:T19)
        n564 = xnode "Read/Write Control"("FPGA VI Reference In"=w923, "error in"=w919, "Direct RF Box  Communication"=FALSE) -> ("FPGA VI Reference Out"=w922:T19, "error out"=w921:errorcluster)
        n565 = flat-sequence {
          tunnel: w921 -> [w952]
          tunnel: [w952] -> w920
          frame #0 {
            n566 = Wait (ms)(milliseconds to wait=u32 50) -> ()  [unwired: 1 out]
          }
        }
        n567 = xnode "Read/Write Control"("FPGA VI Reference In"=w922, "error in"=w920, "FPGA Controls  RF Box"=TRUE) -> ("error out"=w915:errorcluster)  [unwired: 1 out]
        n568 = property on="Restart RF" class="Bool (strict)"(error in=w915, "Value"=FALSE ("Restart RF")) -> (error out=w914:errorcluster)  [unwired: 1 in, 1 out]
      }
      event "Round T2 X": Value Change {
        n569 = event-data() -> ()  [unwired: 7 out]
        n570 = local read "BD 1 Frequency 2 (MHz)"() -> (w955:dbl)
        n571 = Round To Nearest(number=w955) -> (nearest integer value=w954:dbl)
        n572 = property on="BD 1 Frequency 2 (MHz)" class="DigNum (strict)"("Val(Sgnl)"=w954) -> ()  [unwired: 2 in, 2 out]
      }
      event "Stop All": Value Change {
        n573 = event-data() -> ()  [unwired: 7 out]
        n574 = call "hamilton_controller.vi"("action"=T20."DISCONNECT") -> ()  [unwired: 10 in, 1 out]
        n575 = local read "Stop All"() -> (w958:bool)
      }
      event "Delayed Interlace Start": Value Change {
        n576 = event-data() -> ()  [unwired: 7 out]
        n577 = flat-sequence {
          frame #0 {
            n578 = Multiply(x="Delay to Interlace (s)", y=1000.0) -> (x*y=w961:dbl)
            n579 = Wait (ms)(milliseconds to wait=w961) -> ()  [unwired: 1 out]
          }
          frame #1 {
            n580 = property on="Green laser mode" class="RadioBtnsControl (strict)"("Val(Sgnl)"=enum32{"Laser ON", "Laser OFF", "Interlace"}."Interlace" ("Value (Signaling)")) -> ()  [unwired: 2 in, 2 out]
          }
        }
      }
      event "BD 1 Amplitude 1 (%)", "BD 1 Amplitude 2 (%)", "BD 1 Amplitude 3 (%)", "BD 2 Amplitude 1 (%)", "BD 2 Amplitude 2 (%)", "BD 2 Amplitude 3 (%)", "Trap 1 ON", "Trap 2 ON", "Trap 3 ON", "Feedback On/Off", "All FB On/Off": Value Change {
        w985 = i16 1 ("f")
        n581 = event-data() -> ()  [unwired: 7 out]
        n582 = local write "Trap 1 (ON/OFF)"("Trap 1 ON") -> ()
        n583 = local write "Trap 2 (ON/OFF)"("Trap 2 ON") -> ()
        n584 = Boolean To (0,1)(Boolean="Trap 3 ON") -> (0, 1=w986:i16)
        n585 = Boolean To (0,1)(Boolean="Trap 1 ON") -> (0, 1=w987:i16)
        n586 = Boolean To (0,1)(Boolean="Trap 2 ON") -> (0, 1=w988:i16)
        n587 = Select(t=w988, s="Trap ON/OFF X or Y Amp?", f=w985) -> (s? t:f=w983:i16)
        n588 = Select(t=w987, s="Trap ON/OFF X or Y Amp?", f=w985) -> (s? t:f=w984:i16)
        n589 = Select(t=w986, s="Trap ON/OFF X or Y Amp?", f=w985) -> (s? t:f=w982:i16)
        n590 = Select(t=w985, s="Trap ON/OFF X or Y Amp?", f=w988) -> (s? t:f=w980:i16)
        n591 = Select(t=w985, s="Trap ON/OFF X or Y Amp?", f=w987) -> (s? t:f=w981:i16)
        n592 = Select(t=w985, s="Trap ON/OFF X or Y Amp?", f=w986) -> (s? t:f=w979:i16)
        n593 = And(x="All FB On/Off", y="Feedback On/Off") -> (x .and. y?=w977:cluster{"Set 1":bool, "Set 2":bool})
        n594 = local read "BD 1 Amplitude 1 (%)"() -> (w997:dbl)
        n595 = local read "BD 1 Amplitude 2 (%)"() -> (w996:dbl)
        n596 = local read "BD 1 Amplitude 3 (%)"() -> (w995:dbl)
        n597 = Unbundle By Name(w977) -> ("Set 1"=w972:bool, "Set 2"=w969:bool)
        n598 = local read "Y RF Amplitude Limits (%)"() -> (w965:T16)
        n599 = local read "X RF Amplitude Limits (%)"() -> (w966:T16)
        n600 = local read "BD 2 Amplitude 1 (%)"() -> (w998:dbl)
        n601 = local read "BD 2 Amplitude 2 (%)"() -> (w999:dbl)
        n602 = local read "BD 2 Amplitude 3 (%)"() -> (w1000:dbl)
        n603 = And(x="Trap 2 ON", y=w969) -> (x .and. y?=w967:bool)
        n604 = And(x="Trap 1 ON", y=w972) -> (x .and. y?=w970:bool)
        n605 = Multiply(x=w984, y=w997) -> (x*y=w992:dbl)
        n606 = Multiply(x=w996, y=w983) -> (x*y=w990:dbl)
        n607 = Multiply(x=w995, y=w982) -> (x*y=w991:dbl)
        n608 = Multiply(x=w998, y=w981) -> (x*y=w1001:dbl)
        n609 = Multiply(x=w999, y=w980) -> (x*y=w1002:dbl)
        n610 = Multiply(x=w1000, y=w979) -> (x*y=w1003:dbl)
        n611 = call "set RF board amplitude - interlace.vi"("Board 2 Amplitude Limits"=w965, "Board 1 Amplitude Limits"=w966, "error in"=w993, "FPGA VI Reference In"=w994, "Board 2 Amplitude 3 (%)"=w1003, "Board 1 Amplitude 3 (%)"=w991, "Board 2 Amplitude 2 (%)"=w1002, "Board 2 Amplitude 1 (%)"=w1001, "Board 1 Amplitude 2 (%)"=w990, "Board 1 Amplitude 1 (%)"=w992) -> ("error out"=w974:errorcluster, "FPGA VI Reference Out"=w975:T19)
        n612 = xnode "Read/Write Control"("FPGA VI Reference In"=w975, "error in"=w974, "FB On/Off Set 1"=w970, "FB On/Off Set 2"=w967) -> ("error out"=w973:errorcluster)  [unwired: 1 out]
      }
      event "Load parameters": Value Change {
        n613 = event-data() -> ()  [unwired: 7 out]
        n614 = property on="Saved AOD Raster Scan Parameter Sets" class="Arr (strict)"() -> ("Index Values"=w1014:u32[])  [unwired: 2 in, 2 out]
        n615 = Index Array(array=w1014, index=0) -> (element=w1011:u32)
        n616 = local write "Load parameters"(FALSE ("Load parameters")) -> ()
        n617 = Index Array(array="Saved AOD Raster Scan Parameter Sets", index=w1011) -> (element=w1010:T30)
        n618 = Unbundle By Name(w1010) -> ("Scan Range AOD (nm) 2"=w1009:dbl, "Step Size AOD (nm) 2"=w1008:dbl, "Scan Speed AOD (nm/s) 2"=w1007:dbl, "Number of scans (AOD) 2"=w1006:u16)
        n619 = flat-sequence {
          tunnel: w1009 -> [w1017]
          tunnel: w1008 -> [w1016]
          tunnel: w1007 -> [w1015]
          tunnel: w1006 -> [w1018]
          frame #0 {
            n620 = local write "Scan Speed (nm/s)"(w1015) -> ()
            n621 = local write "Scan Range (nm)"(w1017) -> ()
            n622 = local write "Step Size (nm)"(w1016) -> ()
          }
          frame #1 {
            n623 = property on="Number of F/B Scans (AOD)" class="DigNum (strict)"("Val(Sgnl)"=w1018) -> ()  [unwired: 2 in, 2 out]
          }
        }
      }
      event "Trap 1 (ON/OFF)", "Trap 2 (ON/OFF)": Value Change {
        n624 = event-data() -> ()  [unwired: 7 out]
        n625 = property on="Trap 2 ON" class="Bool (strict)"("Val(Sgnl)"="Trap 2 (ON/OFF)") -> ()  [unwired: 2 in, 2 out]
        n626 = property on="Trap 1 ON" class="Bool (strict)"("Val(Sgnl)"="Trap 1 (ON/OFF)") -> ()  [unwired: 2 in, 2 out]
      }
      event "DIO count 1 (ticks)", "DIO count 2 (ticks)", "DIO count 3 (ticks)", "Interlace", "Number Interlace Sets", "Not-Interlacing Set": Value Change {
        n627 = event-data() -> ()  [unwired: 7 out]
        n628 = local read "DIO count 3 (ticks)"() -> (w1031:u32)
        n629 = local read "DIO count 1 (ticks)"() -> (w1033:u32)
        n630 = local read "DIO count 2 (ticks)"() -> (w1032:u32)
        n631 = To Unsigned Byte Integer(number="Not-Interlacing Set") -> (unsigned 8bit integer=w1022:u8)
        n632 = Add(x=w1022, y=u8 1) -> (x+y=w1026:u8)
        n633 = xnode "Read/Write Control"("FPGA VI Reference In"=w1037, "error in"=w1035, "DIO count 1 (ticks)"=w1033, "DIO count 2 (ticks)"=w1032, "DIO count 3 (ticks)"=w1031, "Interlace ON/OFF"="Interlace", "Number Interlace Cycles"="Number Interlace Sets", "Interlace Off Parameters"=w1026) -> ("error out"=w1036:errorcluster)  [unwired: 1 out]
        n634 = Build Array(w1033, w1032, w1031) -> (w1024:u32[])
        n635 = Split 1D Array(array=w1024, index="Number Interlace Sets") -> (first subarray=w1034:u32[])  [unwired: 1 out]
        n636 = Index Array(array=w1024, index=w1022) -> (element=w1023:u32)
        n637 = Add Array Elements(numeric array=w1034) -> (sum=w1028:u32)
        n638 = Select(t=w1028, s="Interlace", f=w1023) -> (s? t:f=→"Total Counts (ticks)":u32)
      }
      event "Reset Feedback": Value Change {
        n639 = event-data() -> ()  [unwired: 7 out]
        n640 = Unbundle By Name("Reset Feedback") -> ("Set 1"=w1041:bool, "Set 2"=w1040:bool)
        n641 = xnode "Read/Write Control"("FPGA VI Reference In"=w1043, "error in"=w1038, "FB Reset Set 1"=w1041, "FB Reset Set 2"=w1040) -> ("error out"=w1039:errorcluster)  [unwired: 1 out]
      }
      event "PID Gains": Value Change {
        n642 = event-data() -> ()  [unwired: 7 out]
        n643 = Unbundle By Name("PID Gains") -> ("Set 1"=w1047:T14, "Set 2"=w1046:T14)
        n644 = xnode "Read/Write Control"("FPGA VI Reference In"=w1048, "error in"=w1044, "FB Gains Set 1"=w1047, "FB Gains Set 2"=w1046) -> ("error out"=w1045:errorcluster)  [unwired: 1 out]
      }
      event "AI2 to Setpoint", "Trap Intensity\nSetpoints (V)": Value Change {
        n645 = event-data() -> ()  [unwired: 7 out]
        n646 = xnode "Read/Write Control"("FPGA VI Reference In"=w1054, "error in"=w1050) -> ("FPGA VI Reference Out"=w1053:T19, "error out"=w1052:errorcluster, "AI4 Y Sum Set 1"=w1061:i16, "AI4 Y Sum Set 2"=w1060:i16)
        n647 = Cluster To Array(cluster="AI2 to Setpoint") -> (array=w1064:bool[])
        n648 = local read "AI2 (V)"() -> (w1062:cluster{"Set 1":dbl, "Set 2":dbl})
        n649 = Or Array Elements(Boolean array=w1064) -> (logical OR=w1065:bool)
        n650 = Bundle By Name(cluster=w1062, "Set 1"=w1061, "Set 2"=w1060) -> (w1059:cluster{"Set 1":dbl, "Set 2":dbl})
        n651 = Divide(x=w1059, y=3276.7) -> (x/y=w1058:cluster{"Set 1":dbl, "Set 2":dbl})
        "AI2 (V)" <- w1058
        n652 = case shown="True" w1065 {
          tunnel: [w1068 w1085] -> w1057
          tunnel: "AI2 to Setpoint" -> [_ w1081]
          tunnel: "Trap Intensity\nSetpoints (V)" -> [w1069 w1084]
          tunnel: w1058 -> [_ w1078]
          frame False {
            n653 = Multiply(x=3276.7, y=w1069) -> (x*y=w1070:cluster{"Set 1":dbl, "Set 2":dbl})
            n654 = To Word Integer(number=w1070) -> (16bit integer=w1068:cluster{"Set 1":i16, "Set 2":i16})
          }
          frame True {
            n655 = Unbundle By Name(w1078) -> ("Set 1"=w1077:dbl, "Set 2"=w1076:dbl)
            n656 = Unbundle By Name(w1084) -> ("Set 1"=w1083:dbl, "Set 2"=w1082:dbl)
            n657 = Unbundle By Name(w1081) -> ("Set 1"=w1080:bool, "Set 2"=w1079:bool)
            n658 = Select(t=w1077, s=w1080, f=w1083) -> (s? t:f=w1075:dbl)
            n659 = Select(t=w1076, s=w1079, f=w1082) -> (s? t:f=w1074:dbl)
            n660 = Bundle By Name(cluster=w1084, "Set 1"=w1075, "Set 2"=w1074) -> (w1072:cluster{"Set 1":dbl, "Set 2":dbl})
            n661 = local write "Trap Intensity\nSetpoints (V)"(w1072) -> ()
            n662 = Multiply(x=3276.7, y=w1072) -> (x*y=w1073:cluster{"Set 1":dbl, "Set 2":dbl})
            n663 = To Word Integer(number=w1073) -> (16bit integer=w1085:cluster{"Set 1":i16, "Set 2":i16})
          }
        }
        n664 = Unbundle By Name(w1057) -> ("Set 1"=w1056:i16, "Set 2"=w1055:i16)
        n665 = xnode "Read/Write Control"("FPGA VI Reference In"=w1053, "error in"=w1052, "FB Setpoint Set 1"=w1056, "FB Setpoint Set 2"=w1055) -> ("error out"=w1051:errorcluster)  [unwired: 1 out]
      }
      event "Invert GI": Value Change {
        n666 = event-data() -> ()  [unwired: 7 out]
        n667 = xnode "Read/Write Control"("FPGA VI Reference In"=w1090, "error in"=w1088, "Invert GI"="Invert GI", "Invert GI 2"="Invert GI") -> ("error out"=w1089:errorcluster)  [unwired: 1 out]
      }
      event "Green FB Setpoint (mV)", "Green FB Gains", "Green FB On/Off", "Current When FB OFF (%)", "Green int current ON count adj": Value Change {
        n668 = event-data() -> ()  [unwired: 7 out]
        n669 = local read "Green FB Setpoint (mV)"() -> (w1097:dbl)
        n670 = local read "Current When FB OFF (%)"() -> (w1100:dbl)
        n671 = Multiply(x=w1097, y=3.2767) -> (x*y=w1096:dbl)
        n672 = Multiply(x=w1100, y=655.35) -> (x*y=w1101:dbl)
        n673 = To Unsigned Word Integer(number=w1101) -> (unsigned 16bit integer=w1099:u16)
        n674 = local read "Green int current ON count adj"() -> (w1104:u32)
        n675 = local read "Green FB Gains"() -> (w1103:T14)
        n676 = local read "Green Laser ON/Interlacing"() -> (w1094:bool)
        n677 = local read "Green laser mode"() -> (w1093:enum32{"Laser ON", "Laser OFF", "Interlace"})
        n678 = local read "Green FB On/Off"() -> (w1105:bool)
        n679 = Equal?(x=w1093, y=enum32{"Laser ON", "Laser OFF", "Interlace"}."Interlace") -> (x = y?=w1091:bool)
        n680 = Compound Arithmetic op=AND(w1091, w1105, w1094) -> (w1095:bool)
        n681 = xnode "Read/Write Control"("FPGA VI Reference In"=w1108, "error in"=w1107, "Green FB Setpoint"=w1096, "Green FB On/Off"=w1095, "Current Out"=w1099, "Green int current ON count adj"=w1104, "Green FB Gains"=w1103) -> ("error out"=w1106:errorcluster)  [unwired: 1 out]
      }
      event "Green laser mode", "Green Laser ON/Interlacing": Value Change {
        n682 = event-data() -> ()  [unwired: 7 out]
        n683 = case shown="True" "Green Laser ON/Interlacing" {
          tunnel: "Green laser mode" -> [_ w1122]
